vi "FT10_Unitherm Ask Dialog - Set Load.vi"(10 "Set Load in":T1) -> (2 "Set Load out":bool)   [LabVIEW 2024]
doc: "Verifies user wants to change impedance on Unitherm"
uses:
  Controls/Control_Unitherm Set Load Bool.ctl
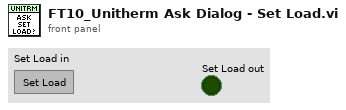
[diagram p1: front panel]
types:
  T1 = typedef "Control_Unitherm Set Load Bool.ctl" = bool
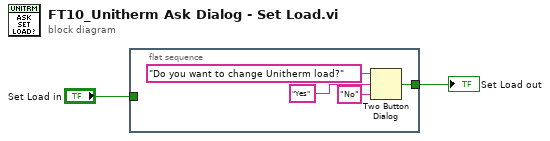
[diagram p0: block diagram]
diagram:
  n1 = flat-sequence {
    tunnel: [w3] -> w2
    tunnel: "Set Load in" -> [_]
    frame #0 {
      n2 = Two Button Dialog(message="Do you want to change Unitherm load?", 1:"No" ("F button name (\"Cancel\")"), 2:"Yes" ("T button name (\"OK\")")) -> (T button?=w3:bool)
    }
  }
  "Set Load out" <- w2
